vi "Form Wire Specs.vi"(8 "error in (no error)":errorcluster, 10 "Not Source Terminals[]":refnum<vi>[](array[refnum]), 11 "Source Terminals":refnum<vi>[](array[refnum])) -> (0 "error out":errorcluster, 3 "Wire Spec":string[][](array[string]))   [LabVIEW 2014]
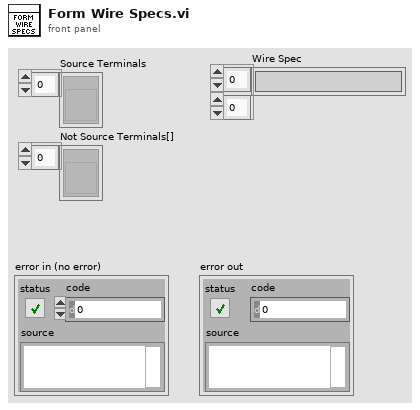
[diagram p1: front panel]
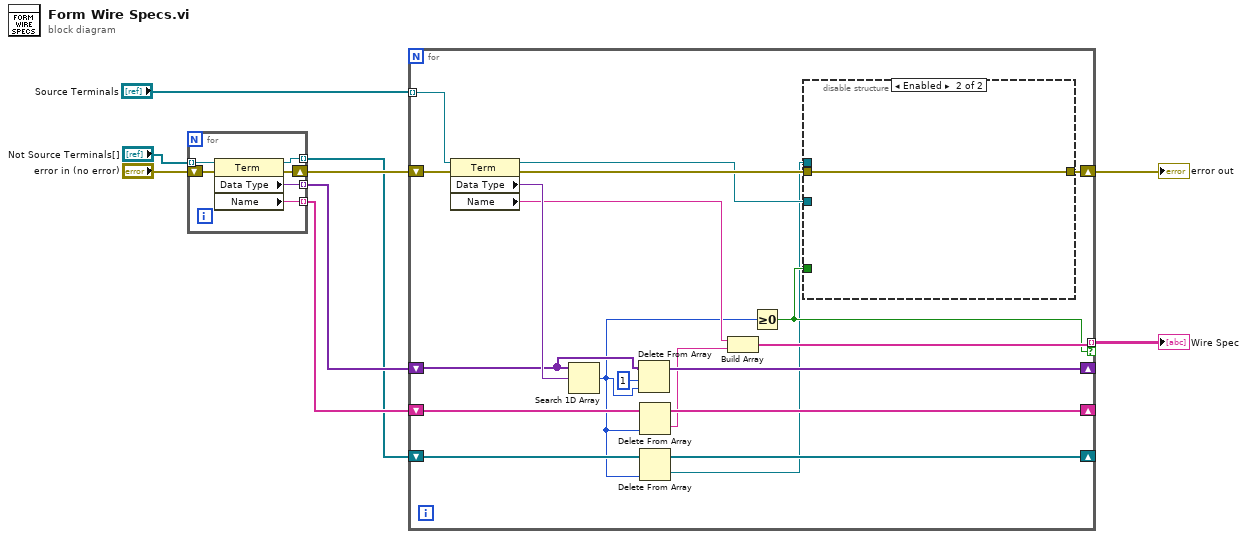
[diagram p0: block diagram]
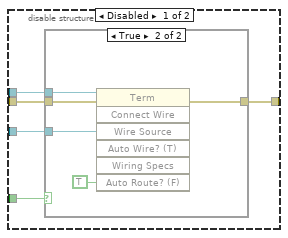
[diagram p2: hidden frame]
diagram:
  n1 = for {
    shift-right: [w14] -> w7
    shift-left: "error in (no error)" -> [w15]
    tunnel: "Not Source Terminals[]" -> [w13] mode=indexing
    tunnel: [w12] -> w4 mode=indexing
    tunnel: [w11] -> w3 mode=indexing
    tunnel: [w10] -> w1 mode=indexing
    n2 = property class="Term"(reference=w13, error in=w15) -> (reference out=w10:refnum<vi>, error out=w14:errorcluster, "Data Type"=w12:variant, "Name"=w11:string)
  }
  n3 = for {
    shift-right: [w22] -> w9
    shift-left: w7 -> [w34]
    tunnel: "Source Terminals" -> [w33] mode=indexing
    shift-right: [w28] -> _
    shift-left: w3 -> [w29]
    shift-right: [w27] -> _
    shift-left: w4 -> [w31]
    tunnel: [w24] -> w2 mode=indexing if=w21
    shift-right: [w18] -> _
    shift-left: w1 -> [w19]
    n4 = property class="Term"(reference=w33, error in=w34) -> (reference out=w20:refnum<vi>, error out=w23:errorcluster, "Data Type"=w32:variant, "Name"=w26:string)
    n5 = Search 1D Array(1D array=w31, element=w32) -> (index of element=w16:i32)  [unwired: 1 in]
    n6 = Delete From Array(array=w31, length=1, index=w16) -> (array with subset deleted=w27:variant[])  [unwired: 1 out]
    n7 = Delete From Array(array=w29, index=w16) -> (deleted portion=w25:string, array with subset deleted=w28:string[])  [unwired: 1 in]
    n8 = Delete From Array(array=w19, index=w16) -> (deleted portion=w17:refnum<vi>, array with subset deleted=w18:refnum<vi>[])  [unwired: 1 in]
    n9 = Build Array(w26, w25) -> (w24:string[])
    n10 = Greater Or Equal To 0?(x=w16) -> (x >= 0?=w21:bool)
    n11 = disable-structure shown="Enabled" {
      disable-tunnel: w23 -> [w39 w46]
      disable-tunnel: [w38 w46] -> w22
      disable-tunnel: w21 -> [w37 _]
      disable-tunnel: w20 -> [w36 _]
      disable-tunnel: w17 -> [w35 _]
      frame Disabled {
        n12 = case shown="True" w37 {
          tunnel: w39 -> [w40 w45]
          tunnel: [w40 w44] -> w38
          tunnel: w36 -> [_ w43]
          tunnel: w35 -> [_ w42]
          frame False {
          }
          frame True {
            n13 = invoke class="Term" method="Connect Wire"(reference=w42, error in=w45, "Wire Source"=w43, "Auto Route? (F)"=TRUE) -> (error out=w44:errorcluster)  [unwired: 3 in, 6 out]
          }
        }
      }
      frame Enabled {
      }
    }
  }
  "error out" <- w9
  "Wire Spec" <- w2
